vi "Trend Estimation (Curve Fitting).vi"() -> ()   [LabVIEW 2023]
doc: "This example shows how to remove a trend from a univariate time series with the TSA Detrend VI.\n\n<b>Instructions:</b>\n1) Run this VI.\n2) Select method to estimate trend and observe the trend and the signal with trend removed."
uses:
  <vilib>/addons/Time Series Analysis/Utilities.llb/TSA Data.ctl
  <vilib>/addons/Time Series Analysis/Series Preprocess.llb/TSA Detrend (Waveform).vi
  <vilib>/addons/_Advanced Signal Processing/NI_AdvSigProcTSA.lvlib
panel:
  in  "Method":u16(ring) items=["Linear", "Quadratic", "Cubic", "N-polynomial", "Exponential"]
  in  "stop":bool
  out "Period Product Sales With Trend Removed":waveform(dbl)(graph)
  out "Period Product Sales":waveform(dbl)[](graph)
  # "Overview: Shows how to remove a trend from a univariate time series with the TSA Detrend VI.\nRequirements: LabVIEW Full Development System, Advanced Signal Processing Toolkit\nInstructions: \n1. Run this VI.\n2. Select method to estimate trend and observe the trend and the signal with trend removed.\n3.  Click Stop to stop the VI."
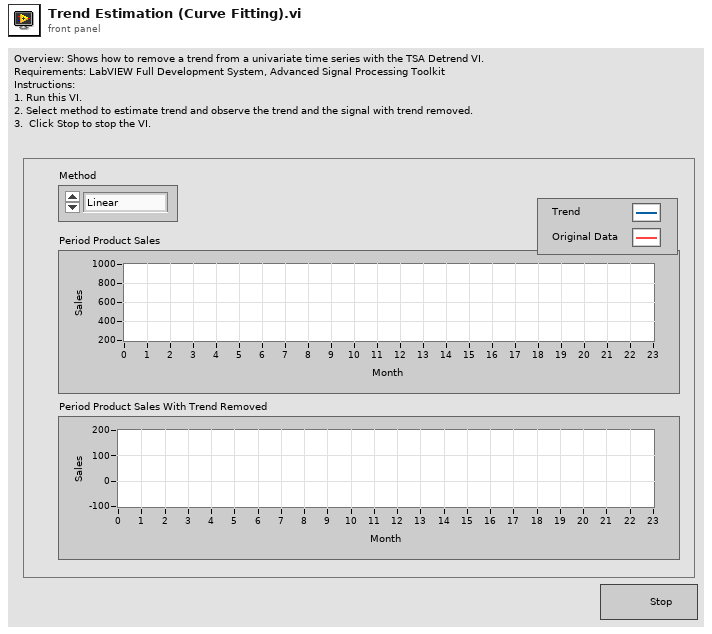
[diagram p1: front panel]
types:
  T1 = typedef "NI_AdvSigProcTSA.lvlib/TSA Data.ctl" = u16
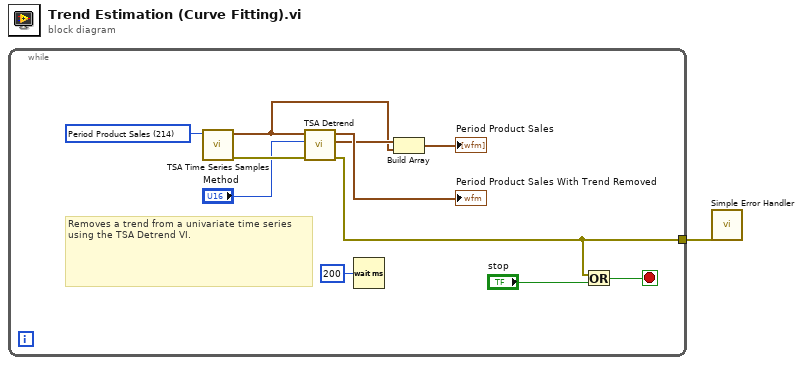
[diagram p0: block diagram]
diagram:
  n1 = while {
    tunnel: [w2] -> w1
    stop <- w6 stop-if-true
    w4 = T1 214 items=["Kobe Earthquake"=201, "EEG"=210, "Bearing Vibration (simulated)"=211, "Period Product Sales"=214, "Beam Vibration (nonlinear)"=217, "Beam Vibration (linear)"=218, "Signal With Echo"=219, "Engine Knocking"=220, "Power Line"=221, "-"=200, "Beam Deflections (multivariate)"=207, "Structure Vibration (multivariate)"=208, "Human MEG (multivariate)"=222] ("data")
    # "Removes a trend from a univariate time series using the TSA Detrend VI."
    n2 = call <vilib>:"TSA Time Series Samples.vi"("data"=w4) -> ("error out"=w11:errorcluster, "univariate time series"=w8:waveform(dbl))  [unwired: 1 in, 8 out]
    n3 = call-poly <vilib>:"TSA Detrend.vi"("error in (no error)"=w11, "method"="Method", "Xt"=w8) -> ("error out"=w2:errorcluster, "trend"=w9:waveform(dbl), "Xt detrended"=→"Period Product Sales With Trend Removed":waveform(dbl))  [unwired: 6 out]
    n4 = Wait (ms)(milliseconds to wait=u32 200 ("millisecond multiple")) -> ()  [unwired: 1 out]
    n5 = Build Array(w9, w8) -> (→"Period Product Sales":waveform(dbl)[])
    n6 = Or(x=w2, y="stop") -> (x .or. y?=w6:bool)
  }
  n7 = call <vilib>:"Simple Error Handler.vi"("error in (no error)"=w1) -> ()  [unwired: 1 in, 8 out]
